vi "DiffKinematics_toWheelSpeed.vi"(9 "CHASSIS Speed":T2 {"vOmega" format="%10.3f"; "vY" format="%10.3f"; "vX" format="%10.3f"}, 11 "DIFF_DRIVE_KINEMATICS":T1 {"TrackWidth_Meters" format="%20.4f"}) -> (1 "RightVelocity":dbl, 3 "LeftVelocity":dbl)   [LabVIEW 2019, in "Trajectory_Library.lvlib"]
doc: "Returns left and right component velocities from a chassis speed using inverse kinematics.\n\nParameters:\n - DiffDriveKinematics - This differential drive kinematics data structure\n - chassisSpeeds - The linear and angular (dx and dtheta) components that represent the chassis' speed.\n\nReturns:\n - LeftVelocity - Left wheel velocity (meters/sec )\n - RightVelocity - Right wheel velocity (meters/sec)"
uses:
  Trajectory_Library.lvlib
  TypeDef/CHASSIS_SPEEDS.ctl
  TypeDef/DIFF_DRIVE_KINEMATICS.ctl
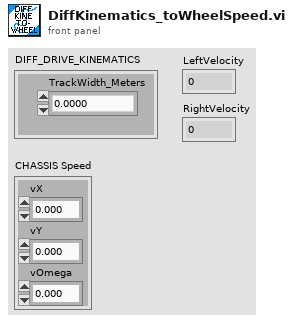
[diagram p1: front panel]
types:
  T1 = typedef "Trajectory_Library.lvlib/DIFF_DRIVE_KINEMATICS.ctl" = cluster{"TrackWidth_Meters":dbl}
  T2 = typedef "Trajectory_Library.lvlib/CHASSIS_SPEEDS.ctl" = cluster{"vX":dbl, "vY":dbl, "vOmega":dbl}
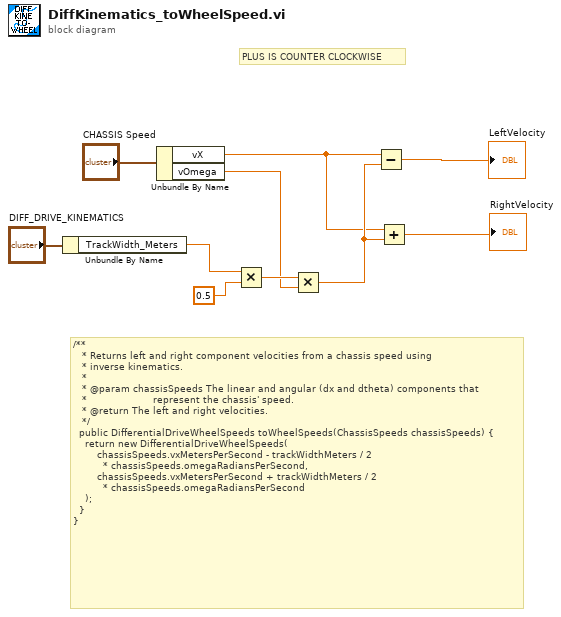
[diagram p0: block diagram]
diagram:
  # "PLUS IS COUNTER CLOCKWISE"
  # "/**\n   * Returns left and right component velocities from a chassis speed using\n   * inverse kinematics.\n   *\n   * @param chassisSpeeds The linear and angular (dx and dtheta) components that\n   *                      represent the chassis' speed.\n   * @return The left and right velocities.\n   */\n  public DifferentialDriveWheelSpeeds toWheelSpeeds(ChassisSpeeds chassisSpeeds) {\n    return new DifferentialDriveWheelSpeeds(\n        chassisSpeeds.vxMetersPerSecond - trackWidthMeters / 2\n          * chassisSpeeds.omegaRadiansPerSecond,\n        chassisSpeeds.vxMetersPerSecond + trackWidthMeters / 2\n          * chassisSpeeds.omegaRadiansPerSecond\n    );\n  }\n}"
  n1 = Unbundle By Name("DIFF_DRIVE_KINEMATICS") -> ("TrackWidth_Meters"=w1:dbl)
  n2 = Unbundle By Name("CHASSIS Speed") -> ("vX"=w4:dbl, "vOmega"=w3:dbl)
  n3 = Multiply(x=w1, y=0.5) -> (x*y=w9:dbl)
  n4 = Multiply(x=w9, y=w3) -> (x*y=w8:dbl)
  n5 = Subtract(x=w4, y=w8) -> (x-y=→"LeftVelocity":dbl)
  n6 = Add(x=w4, y=w8) -> (x+y=→"RightVelocity":dbl)
